vi "3 Tap 10-Bit.vi"() -> ()   [LabVIEW 2015]
uses:
  <vilib>/eio/EIONode/EIONode.xnode
  <vilib>/rvi/eio/common/nirviEmuTemplateMethod_errors.vi
panel:
  out "Pixels":T1
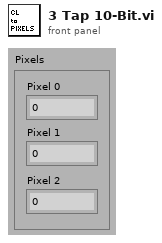
[diagram p1: front panel]
types:
  T1 = cluster{"Pixel 0":u16, "Pixel 1":u16, "Pixel 2":u16}
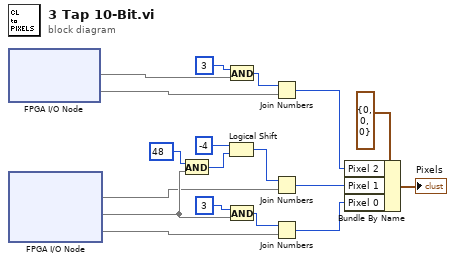
[diagram p0: block diagram]
diagram:
  n1 = xnode "FPGA I/O Node"() -> ("CL Port F"=w4, "CL Port E"=w3)  [unwired: 2 in, 2 out]
  n2 = xnode "FPGA I/O Node"() -> ("CL Port C"=w10, "CL Port B"=w12, "CL Port A"=w11)  [unwired: 3 in, 3 out]
  n3 = And(x=u8 48 ("hi"), y=w12) -> (x .and. y?=w15:u8)
  n4 = Logical Shift(y=i8 -4, x=w15) -> (x << y=w13:u8)
  n5 = And(x=u8 3 ("hi"), y=w4) -> (x .and. y?=w6:u8)
  n6 = And(x=u8 3 ("hi"), y=w12) -> (x .and. y?=w17:u8)
  n7 = Join Numbers(hi=w6, lo=w3) -> ((hi.lo)=w2:u16)
  n8 = Join Numbers(hi=w13, lo=w10) -> ((hi.lo)=w8:u16)
  n9 = Join Numbers(hi=w17, lo=w11) -> ((hi.lo)=w9:u16)
  n10 = Bundle By Name(cluster=T1 {"Pixel 0"=0, "Pixel 1"=0, "Pixel 2"=0} ("PixelData"), "Pixel 2"=w2, "Pixel 1"=w8, "Pixel 0"=w9) -> (→"Pixels":T1)
